vi "Read configuration.vi"(8 "error in":errorcluster, 11 "System Diagnostics editor node in":refnum<class "System Diagnostics editor node.lvclass">) -> (0 "error out":errorcluster, 2 "configuration":refnum<class "NISE_CEF_serializable configuration.lvclass">, 3 "System Diagnostics editor node out":refnum<class "System Diagnostics editor node.lvclass">)   [LabVIEW 2013, in "System Diagnostics editor node.lvclass"]
uses:
  System Diagnostics editor node.lvclass
  <vilib>/NI/Configuration Framework/serializable configuration/NISE_CEF_serializable configuration.lvclass
  System Diagnostics editor node.lvclass/System Diagnostics editor node.ctl
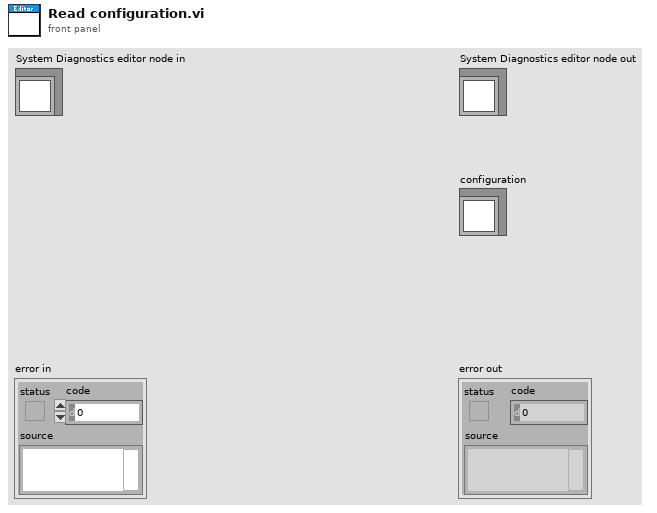
[diagram p1: front panel]
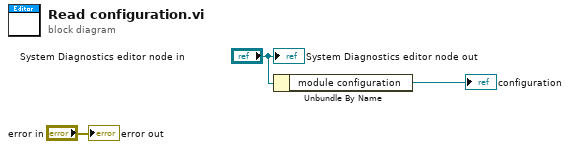
[diagram p0: block diagram]
diagram:
  n1 = Unbundle By Name("System Diagnostics editor node in") -> ("module configuration"=→"configuration":refnum<class "System Diagnostics configuration.lvclass">)
  "error out" <- "error in"
  "System Diagnostics editor node out" <- "System Diagnostics editor node in"
